vi "dvp Vi Get Trigger State.vi"(10 "pTriggerState":i32, 11 "handle":u32) -> (2 "pTriggerState out":i32, 3 "function return":u32(ring))   [LabVIEW 2018, in "LabViewDVPCamera.lvlib"]
doc: "LabviewDvp2Api dvpStatus dvpViGetTriggerState(dvpHandle handle, BOOL *pTriggerState);"
uses:
  LabViewDVPCamera.lvlib
  LabViewDVPCamera/LabViewDVPCamera.dll
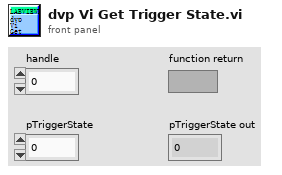
[diagram p1: front panel]
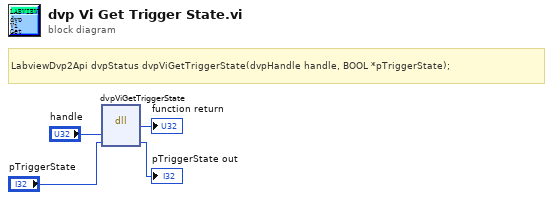
[diagram p0: block diagram]
diagram:
  # "LabviewDvp2Api dvpStatus dvpViGetTriggerState(dvpHandle handle, BOOL *pTriggerState);"
  n1 = dll-call lib="C:/Program Files (x86)/DVP2 Labview cn 64/Sample/LabViewDVPCamera/LabViewDVPCamera.*" fn="dvpViGetTriggerState"("handle"="handle", "pTriggerState"="pTriggerState") -> (→"function return":u32, "pTriggerState"=→"pTriggerState out":i32)  [unwired: 4 in, 2 out]
